vi "Regelung1.vi"() -> ()   [LabVIEW 2010]
panel:
  in  "?":T1(tab)
  out "Waveform Chart":dbl(graph)
  in  "Port":i32(ring) items=["COM 1", "COM 2", "COM 3"]
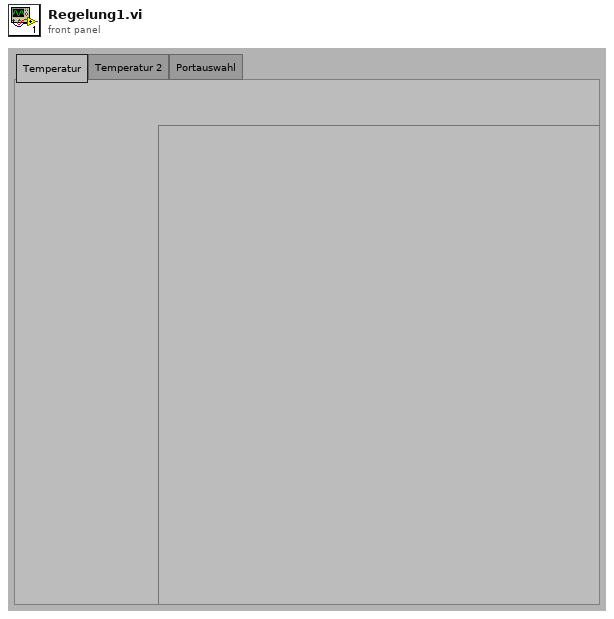
[diagram p1: front panel]
types:
  T1 = enum32{"Temperatur", "Temperatur 2", "Portauswahl"}
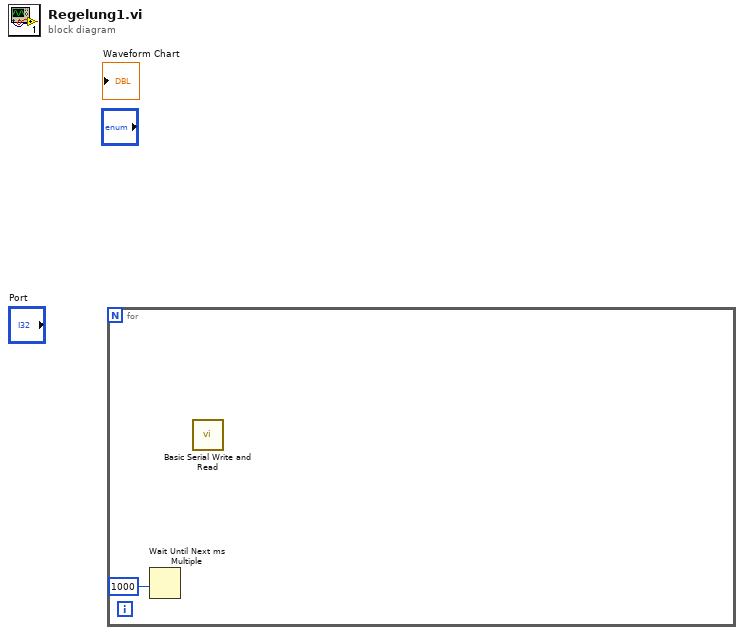
[diagram p0: block diagram]
diagram:
  n1 = for {
    n2 = Wait Until Next ms Multiple(millisecond multiple=u32 1000 ("millisecond timer value")) -> ()  [unwired: 1 out]
    n3 = call "Basic Serial Write and Read.vi"() -> ()  [unwired: 9 in, 2 out]
  }
